vi "Create Client.vi"(0 "Data Holder":T1, 11 "error in (no error)":errorcluster) -> (15 "error out":errorcluster)   [LabVIEW 2021, in "Measurement Client.lvlib"]
uses:
  Measurement Client.lvlib
  Data Holder.ctl
  <vilib>/gRPC/LabVIEW gRPC Library/Shared/grpcId.ctl
  <vilib>/Utility/miscctls.llb/LVPoint32TypeDef.ctl
  <vilib>/Utility/miscctls.llb/LVPositionTypeDef.ctl
  <vilib>/gRPC/LabVIEW gRPC Library/grpc-lvsupport-release.lvlib
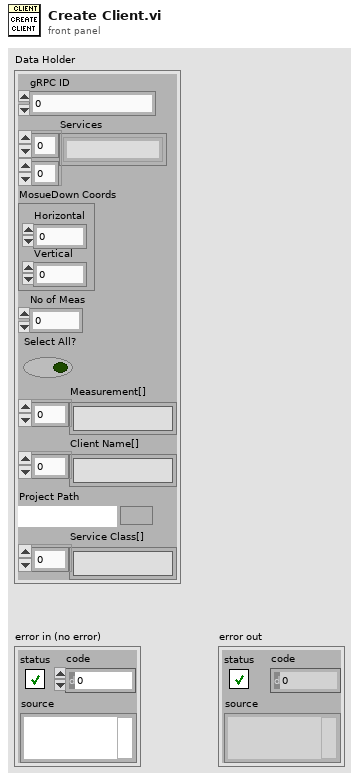
[diagram p1: front panel]
types:
  T1 = typedef "Measurement Client.lvlib/Data Holder.ctl" = cluster{"gRPCid":T2, "Services":string[][], "MosueDown Coords":T3, "No of Meas":i32, "Select All?":bool, "Measurement[]":string[], "Client Name[]":string[], "Project Path":path, "Service Class[]":string[]}
  T2 = typedef "grpc-lvsupport-release.lvlib/grpcId.ctl" = u64
  T3 = typedef "LVPoint32TypeDef.ctl" = cluster{"Horizontal":i32, "Vertical":i32}
  T4 = typedef "LVPositionTypeDef.ctl" = cluster{"Left":i32, "Top":i32}
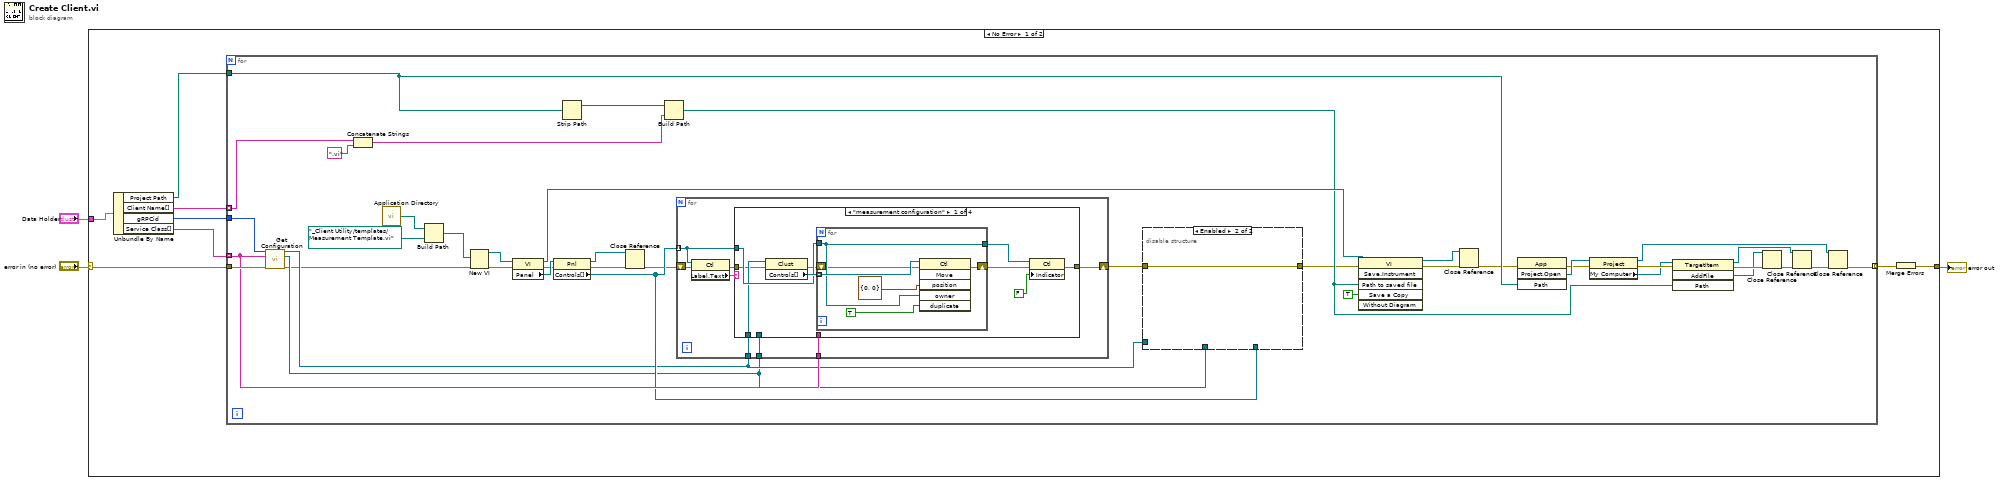
[diagram p0: block diagram]
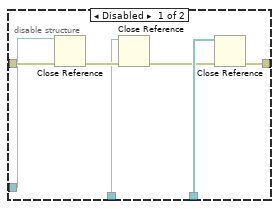
[diagram p2: hidden frame]
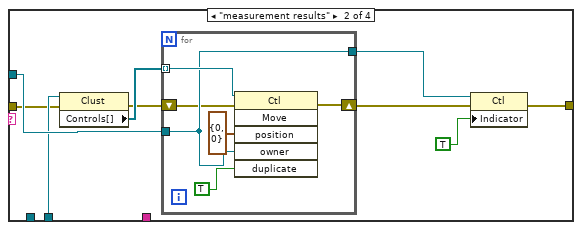
[diagram p3: hidden frame]
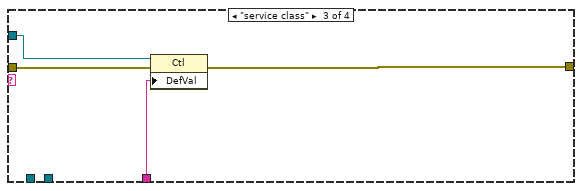
[diagram p4: hidden frame]
diagram:
  n1 = case shown="No Error" "error in (no error)" {
    selector: "error in (no error)" -> [w11 w104]
    tunnel: [w4 w104] -> w3
    tunnel: "Data Holder" -> [w10 _]
    frame No Error {
      n2 = Unbundle By Name(w10) -> ("Project Path"=w7:path, "Client Name[]"=w6:string[], "gRPCid"=w9:T2, "Service Class[]"=w8:string[])
      n3 = for {
        tunnel: w11 -> [w47]
        tunnel: w9 -> [w49]
        tunnel: w8 -> [w45] mode=indexing
        tunnel: w7 -> [w37]
        tunnel: w6 -> [w43] mode=indexing
        tunnel: [w25] -> w5 mode=indexing
        n4 = call "Get Configuration.vi"("gRPCid"=w49, "Service Class"=w45, "error in (no error)"=w47) -> ("Measurement Config"=w19:refnum<vi>, "Measurement Results"=w18:refnum<vi>, "error out"=w12:errorcluster)  [unwired: 10 in]
        n5 = Concatenate Strings(w43, ".vi" ("string")) -> (w41:string)
        n6 = call <vilib>:"Application Directory.vi"() -> ("Application Directory"=w51:path)
        n7 = Build Path(base path=w51, name or relative path=path "_Client Utility/templates/Measurement Template.vi") -> (appended path=w15:path)
        n8 = New VI(8:w12, 10:w15) -> (0:w13:errorcluster, 3:w14:refnum<vi>)  [unwired: 5 in]
        n9 = property class="VI"(reference=w14, error in=w13) -> (reference out=w40:refnum<vi>, error out=w48:errorcluster, "Panel"=w50:refnum<vi>)
        n10 = property class="Pnl"(reference=w50, error in=w48) -> (reference out=w16:refnum<vi>, error out=w46:errorcluster, "Controls[]"=w20:refnum<vi>[])
        n11 = Strip Path(path=w37) -> (stripped path=w44:path)  [unwired: 1 out]
        n12 = Close Reference(reference=w16, error in (no error)=w46) -> (error out=w17:errorcluster)
        n13 = Build Path(base path=w44, name or relative path=w41) -> (appended path=w30:path)
        n14 = for {
          tunnel: w20 -> [w67] mode=indexing
          tunnel: w19 -> [w66]
          tunnel: w18 -> [w65]
          shift-right: [w61] -> w38
          shift-left: w17 -> [w64]
          tunnel: w45 -> [w62]
          n15 = property class="Ctl"(reference=w67, error in=w64) -> (error out=w63:errorcluster, "Label.Text"=w68:string)  [unwired: 1 out]
          n16 = case shown="\"measurement configuration\"" w68 {
            tunnel: w67 -> [w76 w91 w102 _]
            tunnel: w66 -> [w73 _ _ _]
            tunnel: w65 -> [_ w88 _ _]
            tunnel: w63 -> [w72 w87 w101 w103]
            tunnel: w62 -> [_ _ w100 _]
            tunnel: [w69 w84 w99 w103] -> w61
            frame "measurement configuration" {
              n17 = property class="Clust"(reference=w73, error in=w72) -> (error out=w71:errorcluster, "Controls[]"=w77:refnum<vi>[])  [unwired: 1 out]
              n18 = for {
                tunnel: w77 -> [w83] mode=indexing
                tunnel: w76 -> [w80]
                tunnel: [w80] -> w75
                shift-right: [w78] -> w70
                shift-left: w71 -> [w79]
                n19 = invoke class="Ctl" method="Move"(reference=w83, error in=w79, "position"=T4 {"Left"=0, "Top"=0}, "owner"=w80, "duplicate"=TRUE ("Duplicate? (F)")) -> (error out=w78:errorcluster)  [unwired: 1 in, 5 out]
              }
              n20 = property class="Ctl"(reference=w75, error in=w70, "Indicator"=FALSE) -> (error out=w69:errorcluster)  [unwired: 1 out]
            }
            frame "measurement results" {
              n21 = property class="Clust"(reference=w88, error in=w87) -> (error out=w86:errorcluster, "Controls[]"=w92:refnum<vi>[])  [unwired: 1 out]
              n22 = for {
                tunnel: w92 -> [w98] mode=indexing
                tunnel: w91 -> [w95]
                tunnel: [w95] -> w90
                shift-right: [w93] -> w85
                shift-left: w86 -> [w94]
                n23 = invoke class="Ctl" method="Move"(reference=w98, error in=w94, "position"=T4 {"Left"=0, "Top"=0}, "owner"=w95, "duplicate"=TRUE ("Duplicate? (F)")) -> (error out=w93:errorcluster)  [unwired: 1 in, 5 out]
              }
              n24 = property class="Ctl"(reference=w90, error in=w85, "Indicator"=TRUE) -> (error out=w84:errorcluster)  [unwired: 1 out]
            }
            frame "service class" {
              n25 = property class="Ctl"(reference=w102, error in=w101, "DefVal"=w100) -> (error out=w99:errorcluster)  [unwired: 1 out]
            }
            frame Default {
            }
          }
        }
        n26 = disable-structure shown="Enabled" {
          disable-tunnel: w38 -> [w59 w60]
          disable-tunnel: [w58 w60] -> w21
          disable-tunnel: w20 -> [w57 _]
          disable-tunnel: w19 -> [w55 _]
          disable-tunnel: w18 -> [w53 _]
          frame Disabled {
            n27 = Close Reference(reference=w55, error in (no error)=w59) -> (error out=w56:errorcluster)
            n28 = Close Reference(reference=w53, error in (no error)=w56) -> (error out=w54:errorcluster)
            n29 = Close Reference(reference=w57, error in (no error)=w54) -> (error out=w58:errorcluster)
          }
          frame Enabled {
          }
        }
        n30 = invoke class="VI" method="Save.Instrument"(reference=w40, error in=w21, "Path to saved file"=w30, "Save a Copy"=TRUE) -> (reference out=w22:refnum<vi>, error out=w35:errorcluster)  [unwired: 2 in, 4 out]
        n31 = Close Reference(reference=w22, error in (no error)=w35) -> (error out=w23:errorcluster)
        n32 = invoke class="App" method="Project.Open"(error in=w23, "Path"=w37) -> (error out=w34:errorcluster, "Project:Open"=w36:refnum<vi>)  [unwired: 2 in, 2 out]
        n33 = property class="Project"(reference=w36, error in=w34) -> (reference out=w24:refnum<vi>, error out=w33:errorcluster, "My Computer"=w32:refnum<vi>)
        n34 = invoke class="TargetItem" method="AddFile"(reference=w32, error in=w33, "Path"=w30) -> (reference out=w26:refnum<vi>, error out=w31:errorcluster, "AddFile"=w28:refnum<vi>)  [unwired: 1 in, 1 out]
        n35 = Close Reference(reference=w28, error in (no error)=w31) -> (error out=w29:errorcluster)
        n36 = Close Reference(reference=w26, error in (no error)=w29) -> (error out=w27:errorcluster)
        n37 = Close Reference(reference=w24, error in (no error)=w27) -> (error out=w25:errorcluster)
      }
      n38 = Merge Errors(w5) -> (w4:errorcluster)
    }
    frame Error {
    }
  }
  "error out" <- w3
